vi "Filter (G3)-Design.vi"(6 "order":i32=7, 7 "Type":T1 caption="Filter", 8 "Class":enum16{"Elliptic", "Butterworth"}(ring), 9 "low cutoff freq: fl":dbl=0.125 format="%0.3f", 10 "high cutoff freq: fh":dbl=0.45 format="%0.3f", 11 "sampling freq: fs":dbl=1.0 format="%0.2f") -> (0 "error":i32, 3 "IIR Filter":T2)   [LabVIEW 2020]
uses:
  XControls/Filter (G3)/Filter Type.ctl
  <vilib>/Analysis/NI_AALBase.lvlib
  XControls/Filter (G3)/Filter (G3).xctl
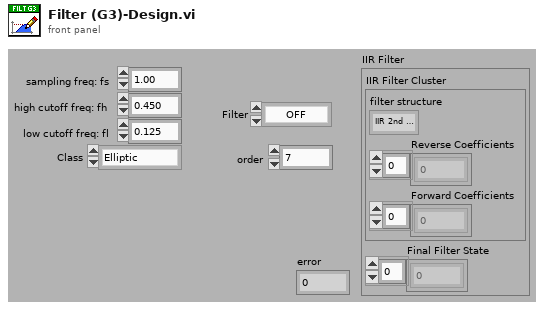
[diagram p1: front panel]
types:
  T1 = typedef "Filter (G3).xctl/Filter Type.ctl" = enum16{"OFF", "Lowpass", "Highpass", "Bandpass", "Bandstop"}
  T2 = cluster{"IIR Filter Cluster":cluster{"filter structure":enum32{"IIR 2nd Order", "IIR 4th Order"}, "Reverse Coefficients":dbl[], "Forward Coefficients":dbl[]}, "Final Filter State":dbl[]}
  T3 = cluster{"filter structure":enum32{"IIR 2nd Order", "IIR 4th Order"}, "Reverse Coefficients":dbl[], "Forward Coefficients":dbl[]}
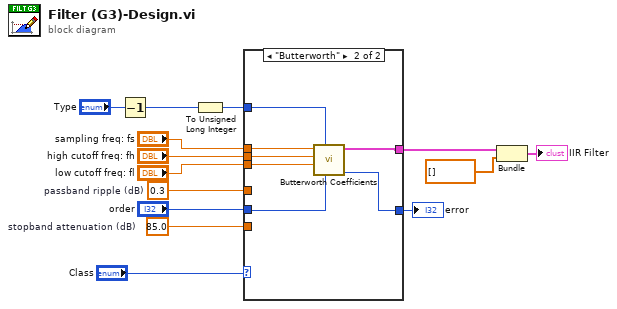
[diagram p0: block diagram]
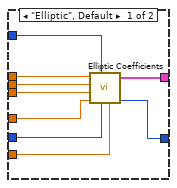
[diagram p2: hidden frame]
diagram:
  w12 = 85.0  # stopband attenuation (dB)
  w14 = 0.3  # passband ripple (dB)
  n1 = Decrement(x="Type") -> (x-1=w2:T1)
  n2 = To Unsigned Long Integer(number=w2) -> (unsigned 32bit integer=w1:u32)
  n3 = case shown="\"Butterworth\"" "Class" {
    tunnel: w14 -> [w23 _]
    tunnel: "order" -> [w22 w27]
    tunnel: w12 -> [w21 _]
    tunnel: w1 -> [w15 w24]
    tunnel: "sampling freq: fs" -> [w20 w30]
    tunnel: "high cutoff freq: fh" -> [w19 w29]
    tunnel: "low cutoff freq: fl" -> [w18 w28]
    tunnel: [w17 w26] -> w8
    tunnel: [w16 w25] -> w4
    frame "Elliptic", Default {
      n4 = call <vilib>:"Elliptic Coefficients.vi"("stopband attenuation (dB)"=w21, "order"=w22, "filter type"=w15, "passband ripple (dB)"=w23, "low cutoff freq: fl"=w18, "high cutoff freq: fh"=w19, "sampling freq: fs"=w20) -> ("error"=w16:i32, "IIR Filter Cluster"=w17:T3)  [unwired: 3 in]
    }
    frame "Butterworth" {
      n5 = call <vilib>:"Butterworth Coefficients.vi"("order"=w27, "filter type"=w24, "low cutoff freq: fl"=w28, "high cutoff freq: fh"=w29, "sampling freq: fs"=w30) -> ("error"=w25:i32, "IIR Filter Cluster"=w26:T3)  [unwired: 5 in]
    }
  }
  "error" <- w4
  n6 = Bundle("IIR Filter Cluster"=w8, "Final Filter State"=dbl[] []) -> (→"IIR Filter":T2)  [unwired: 1 in]
